vi "VerQueryValue.vi"(8 "error in (no error)":errorcluster, 10 "lpSubBlock":string="\\", 11 "lpData":string) -> (0 "error out":errorcluster, 1 "puLen":u32, 2 "lplpBuffer":u64)   [LabVIEW 2013, in "fileversion.lvlib"]
doc: "The VerQueryValue function retrieves specified version information from the version-information resource specified by lpSubBlock. To retrieve the appropriate resource, before you call VerQueryValue, you must first call the GetFileVersionInfoSize function, and then the GetFileVersionInfo function."
uses:
  fileversion.lvlib
  version.dll
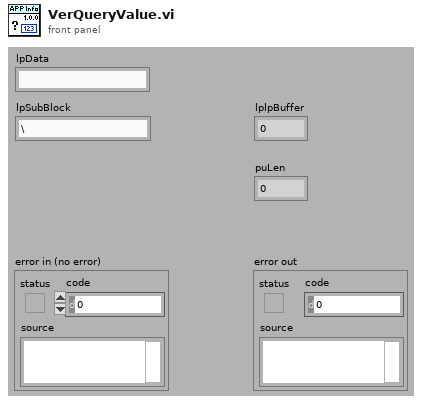
[diagram p1: front panel]
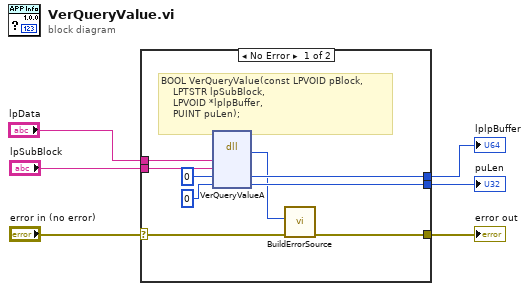
[diagram p0: block diagram]
diagram:
  n1 = case shown="No Error" "error in (no error)" {
    selector: "error in (no error)" -> [w8 w16]
    tunnel: [w7 w16] -> w6
    tunnel: [w13 _] -> w5
    tunnel: [w12 _] -> w4
    tunnel: "lpData" -> [w11 _]
    tunnel: "lpSubBlock" -> [w10 _]
    frame No Error {
      # "BOOL VerQueryValue(const LPVOID pBlock,\n    LPTSTR lpSubBlock,\n    LPVOID *lplpBuffer,\n    PUINT puLen);"
      n2 = dll-call lib="version.dll" fn="VerQueryValueA"("pBlock"=w11, "lpSubBlock"=w10, "lplpBuffer"=u64 0, "puLen"=u32 0) -> ("return type"=w9:i32, "lplpBuffer"=w12:u64, "puLen"=w13:u32)  [unwired: 5 in, 2 out]
      n3 = call "BuildErrorSource.vi"("error in"=w8, "status code"=w9) -> ("error out"=w7:errorcluster)  [unwired: 9 in]
    }
    frame Error {
    }
  }
  "error out" <- w6
  "puLen" <- w5
  "lplpBuffer" <- w4
